vi "Cal11-RunMeasurement.vi"(0 "String in":refnum<vi>, 1 "reference in":refnum<vi>, 2 "Results file output":path, 3 "Array 5":dbl[](array[numeric]), 4 "Array 10":dbl[](array[numeric]), 6 "Array in":dbl[](array[numeric]), 7 "Array 6":dbl[](array[numeric]), 8 "data mode":enum16{"Take new data point", "Refit Curve"}(ring), 9 "Array 11":dbl[](array[numeric]), 11 "-ve Ref Values":bool) -> (10 "Array 8":dbl[](array[numeric]), 12 "Array 7":dbl[](array[numeric]), 13 "Status Out":T1, 14 "Array 9":dbl[](array[numeric]), 15 "Array 4":dbl[](array[numeric]), 16 "Array 3":dbl[](array[numeric]), 17 "String":string, 18 "Sample of input signals":dbl[][](graph))   [LabVIEW 2016]
uses:
  Anemometry Sub Vis/Gen Trav/Multi_Run_Status.ctl
  Anemometry Sub Vis/Controls/Setup.ctl
  Anemometry Sub Vis/Controls/Post_Process.ctl
  Anemometry Sub Vis/Controls/Save_Data.ctl
  <vilib>/Analysis/baseanly.llb/Mean (DBL).vi
  Anemometry Sub Vis/Globals/Calib_global.vi
  Anemometry Sub Vis/Globals/Meas_global.vi
  Anemometry Sub Vis/Acquisition/PWA/PWAtasksGLOBAL.vi
  <vilib>/Analysis/NI_AALBase.lvlib
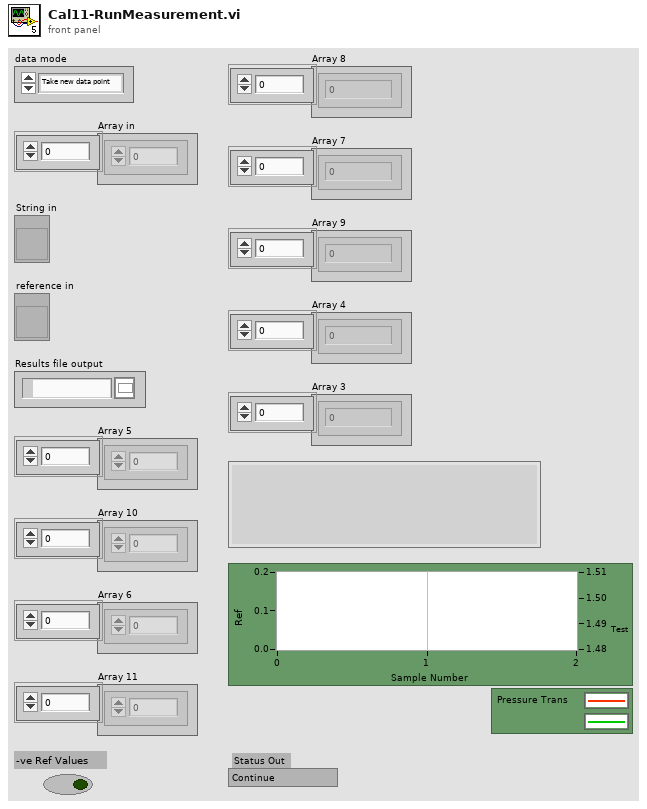
[diagram p1: front panel]
types:
  T1 = typedef "Multi_Run_Status.ctl" = enum16{"Continue", "Jump to Next Point", "Jump to Next Row", "Jump To Fall Back", "Terminate Run"}
  T2 = typedef "Cal_Inst_type.ctl" = enum16{"Propeller anemometer", "Pressure Transducer", "Hot wire", "Cross wire velocity", "Cross wire angle", "Generic Linear", "Generic Polynomial", "Generic BackPoly", "Fast FID", "Thermocouple", "Cold wire", "Pulsed Wire"}
  T3 = typedef "Ref_Inst_type.ctl" = enum16{"Propellor anemometer", "Pressure Transducer", "Raw voltage", "Pitot-static tube", "Preston tube", "Generic Linear", "Generic Polynomial", "Thermocouple", "LDA", "Enter Value", "ADAM Channel"}
  T4 = cluster{"2nd Ref type":T3, "2nd inst present":bool}
  T5 = typedef "Save_Data.ctl" = enum16{"Save No Data", "Save Data"}
  T6 = typedef "Post_Process.ctl" = enum16{"Take New Data", "Post Process Raw Data File"}
  T7 = typedef "Setup.ctl" = enum16{"Run Program", "Show Setup", "Save Current Setup", "Setup Front Panel"}
  T8 = typedef "Analysis_info_cluster.ctl" = cluster{"Colour":u32, "Inst type":T9, "Inst name":string, "Symbol":string, "Code name":string, "Extra Info":string, "Inst Array":T10, "Extra Titles":string[], "Extra Values":string[], "U":dbl, "u^2":dbl, "u^3":dbl, "u^4":dbl, "Skew_u":dbl, "Kurt_u":dbl, "Sd Error in Mean":dbl, "% u'/U":dbl, "X":dbl, "Y":dbl, "Z":dbl, "Timescale integral Estimate":dbl, "Sd Error in Variance":dbl, "Calib File":path, "Calib Constants":dbl[], "Output Position":bool, "Full Stats":bool, "Av Sampling Rate":dbl, "Av No of Samples":dbl, "Total Meas Time (s)":dbl, "ADAM Ch Name":string, "Max value":dbl, "Min value":dbl}
  T9 = typedef "Inst_type.ctl" = enum16{"Propeller anemometer", "Raw voltage", "Pressure Transducer", "Pitot-static tube", "Preston tube", "Hot wire", "Cross wire 1", "Cross wire 2", "Generic Linear", "Generic Polynomial", "Generic BackPoly", "Fast FID", "Thermocouple", "Cold wire", "Pulsed Wire", "LDA Vel", "LDA Tran time", "LDA Arr time", "Microphone"}
  T10 = typedef "Instrument_Array.ctl" = enum16{"PWA", "LDA", "Analogue"}
  T11 = typedef "Time_Trace_Cluster.ctl" = cluster{"Weighting":dbl[], "Time (s)":dbl[], "Voltage":dbl[], "Eng Values":dbl[]}
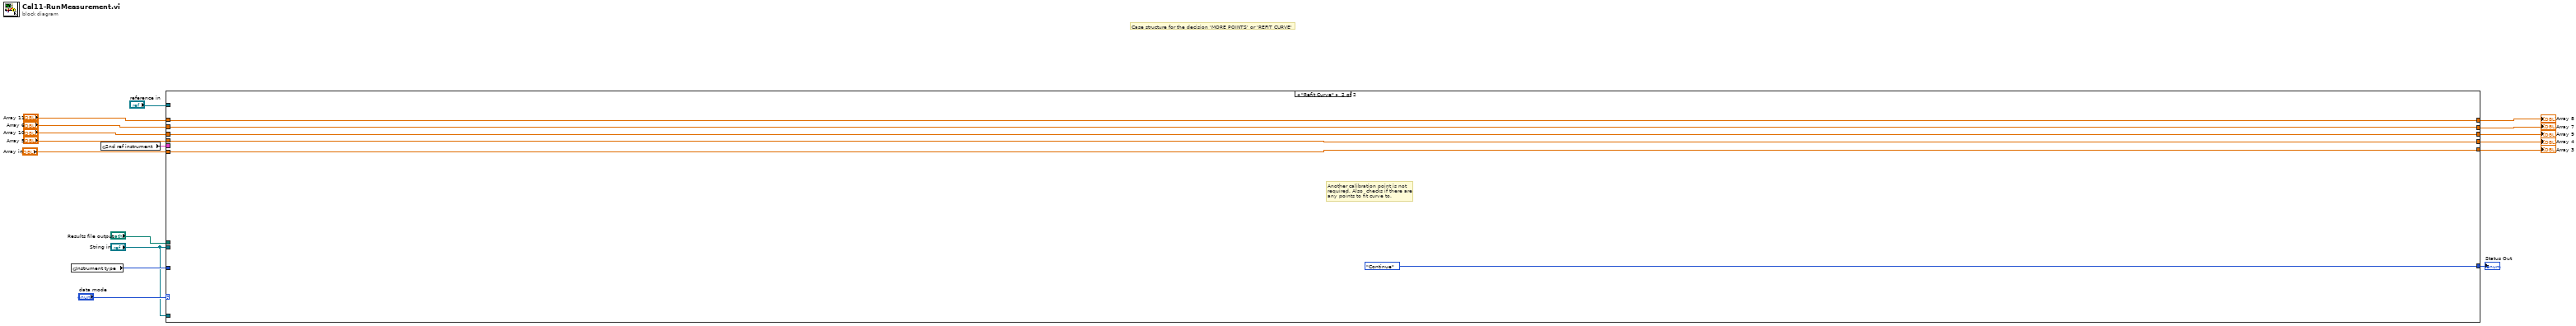
[diagram p0: block diagram]
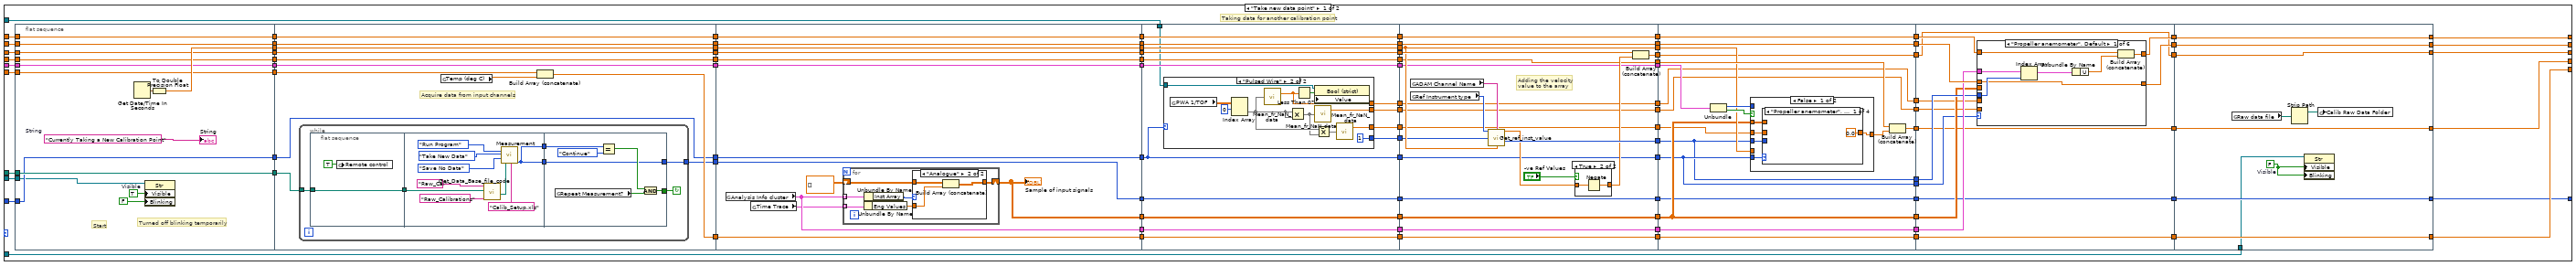
[diagram p2: hidden frame]
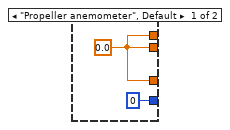
[diagram p4: hidden frame]
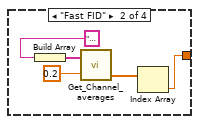
[diagram p6: hidden frame]
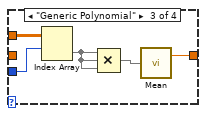
[diagram p7: hidden frame]
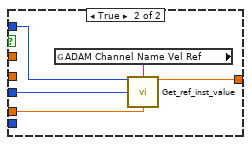
[diagram p9: hidden frame]
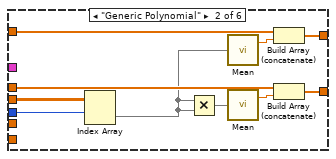
[diagram p10: hidden frame]
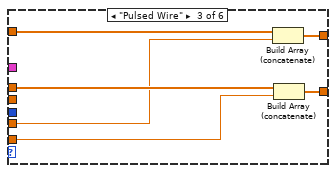
[diagram p11: hidden frame]
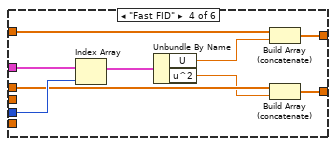
[diagram p12: hidden frame]
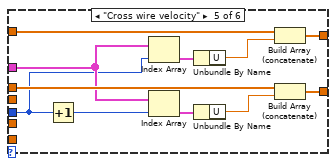
[diagram p13: hidden frame]
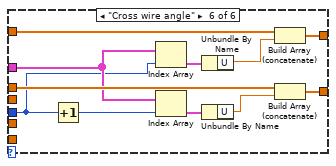
[diagram p14: hidden frame]
diagram:
  # "Case structure for the decision 'MORE POINTS' or 'REFIT CURVE'"
  n1 = global read "Calib_global.vi" "Instrument type"() -> (w16:T2)
  n2 = global read "Calib_global.vi" "2nd ref instrument"() -> (w11:T4)
  n3 = case shown="\"Refit Curve\"" "data mode" {
    tunnel: [w108 w362] -> w6
    tunnel: [w109 w358] -> w5
    tunnel: "Array 11" -> [w110 w362]
    tunnel: "Array 10" -> [w111 w358]
    tunnel: [w107 w361] -> w7
    tunnel: "Array 6" -> [w106 w361]
    tunnel: "Array 5" -> [w105 w360]
    tunnel: [w103 w360] -> w10
    tunnel: w11 -> [w104 _]
    tunnel: [w101 w359] -> w12
    tunnel: "Array in" -> [w102 w359]
    tunnel: "Results file output" -> [w100 _]
    tunnel: [w99 Multi_Run_Status."Continue" ("Status Out")] -> w13
    tunnel: w16 -> [w98 _]
    tunnel: "String in" -> [w20 _]
    tunnel: "reference in" -> [w19 _]
    tunnel: "String in" -> [w18 _]
    frame "Take new data point" {
      # "Taking data for another calibration point"
      # "Start"
      n4 = flat-sequence {
        tunnel: w110 -> [w122]
        tunnel: [w122] -> w97
        tunnel: w111 -> [w121]
        tunnel: [w121] -> w96
        tunnel: w106 -> [w120]
        tunnel: [w120] -> w95
        tunnel: w105 -> [w119]
        tunnel: [w119] -> w94
        tunnel: w104 -> [w118]
        tunnel: [w118] -> w93
        tunnel: w102 -> [w117]
        tunnel: [w117] -> w92
        tunnel: w100 -> [w116]
        tunnel: [w116] -> w91
        tunnel: w98 -> [w115]
        tunnel: [w115] -> w90
        tunnel: [w125] -> w89
        tunnel: w20 -> [w113]
        tunnel: w97 -> [w132]
        tunnel: [w132] -> w88
        tunnel: w96 -> [w131]
        tunnel: [w131] -> w87
        tunnel: w95 -> [w130]
        tunnel: [w130] -> w86
        tunnel: w94 -> [w129]
        tunnel: [w129] -> w85
        tunnel: w93 -> [w128]
        tunnel: [w128] -> w84
        tunnel: w92 -> [w137]
        tunnel: [w136] -> w83
        tunnel: w91 -> [w134]
        tunnel: [w135] -> w82
        tunnel: w90 -> [w127]
        tunnel: [w127] -> w81
        tunnel: w89 -> [w126]
        tunnel: [w126] -> w80
        tunnel: w88 -> [w170]
        tunnel: [w170] -> w79
        tunnel: w87 -> [w169]
        tunnel: [w169] -> w78
        tunnel: w86 -> [w168]
        tunnel: [w168] -> w77
        tunnel: w85 -> [w167]
        tunnel: [w167] -> w76
        tunnel: w84 -> [w166]
        tunnel: [w166] -> w75
        tunnel: w83 -> [w165]
        tunnel: [w165] -> w74
        tunnel: w82 -> [w164]
        tunnel: [w164] -> w73
        tunnel: w81 -> [w163]
        tunnel: [w163] -> w72
        tunnel: w80 -> [w162]
        tunnel: [w162] -> w71
        tunnel: [w173] -> w70
        tunnel: [w161] -> w69
        tunnel: w79 -> [w195]
        tunnel: [w195] -> w68
        tunnel: w78 -> [w194]
        tunnel: [w194] -> w67
        tunnel: w77 -> [w193]
        tunnel: [w193] -> w66
        tunnel: w76 -> [w192]
        tunnel: [w192] -> w65
        tunnel: w75 -> [w191]
        tunnel: [w191] -> w64
        tunnel: w74 -> [w190]
        tunnel: [w190] -> w63
        tunnel: w73 -> [w189]
        tunnel: [w189] -> w62
        tunnel: w72 -> [w198]
        tunnel: [w198] -> w61
        tunnel: w71 -> [w188]
        tunnel: [w188] -> w60
        tunnel: w70 -> [w187]
        tunnel: [w187] -> w59
        tunnel: w69 -> [w186]
        tunnel: [w186] -> w58
        tunnel: [w199] -> w57
        tunnel: [w197] -> w56
        tunnel: [w196] -> w55
        tunnel: [w185] -> w54
        tunnel: w19 -> [w184]
        tunnel: w68 -> [w224]
        tunnel: [w224] -> w53
        tunnel: [w234] -> w52
        tunnel: w67 -> [w233]
        tunnel: w66 -> [w223]
        tunnel: [w223] -> w51
        tunnel: w65 -> [w222]
        tunnel: [w222] -> w50
        tunnel: w64 -> [w221]
        tunnel: [w221] -> w49
        tunnel: w63 -> [w220]
        tunnel: [w220] -> w48
        tunnel: w62 -> [w219]
        tunnel: [w219] -> w47
        tunnel: w61 -> [w218]
        tunnel: [w218] -> w46
        tunnel: [w231] -> w45
        tunnel: w60 -> [w232]
        tunnel: [w232] -> w44
        tunnel: w59 -> [w217]
        tunnel: [w217] -> w43
        tunnel: w58 -> [w216]
        tunnel: [w216] -> w42
        tunnel: w57 -> [w227]
        tunnel: w56 -> [w215]
        tunnel: [w215] -> w41
        tunnel: w55 -> [w214]
        tunnel: [w214] -> w40
        tunnel: w54 -> [w213]
        tunnel: [w213] -> w39
        tunnel: w53 -> [w246]
        tunnel: [w246] -> w38
        tunnel: w52 -> [w245]
        tunnel: [w245] -> w37
        tunnel: w51 -> [w244]
        tunnel: [w244] -> w36
        tunnel: w50 -> [w253]
        tunnel: [w252] -> w35
        tunnel: w49 -> [w251]
        tunnel: w48 -> [w243]
        tunnel: [w243] -> w34
        tunnel: w47 -> [w239]
        tunnel: [w239] -> w33
        tunnel: w46 -> [w248]
        tunnel: [w248] -> w32
        tunnel: w45 -> [w238]
        tunnel: w44 -> [w250]
        tunnel: w43 -> [w242]
        tunnel: [w242] -> w31
        tunnel: [w238] -> w30
        tunnel: w42 -> [w249]
        tunnel: [w249] -> w29
        tunnel: w41 -> [w241]
        tunnel: [w241] -> w28
        tunnel: w40 -> [w240]
        tunnel: [w240] -> w27
        tunnel: w39 -> [w247]
        tunnel: w38 -> [w292]
        tunnel: w37 -> [w282]
        tunnel: [w282] -> w26
        tunnel: [w291] -> w25
        tunnel: [w290] -> w24
        tunnel: w36 -> [w289]
        tunnel: w35 -> [w281]
        tunnel: [w281] -> w23
        tunnel: w34 -> [w280]
        tunnel: [w280] -> w22
        tunnel: w33 -> [w279]
        tunnel: [w279] -> w21
        tunnel: w32 -> [w285]
        tunnel: w31 -> [w288]
        tunnel: w30 -> [w287]
        tunnel: w29 -> [w286]
        tunnel: w28 -> [w284]
        tunnel: w27 -> [w283]
        tunnel: [w354] -> w109
        tunnel: w26 -> [w354]
        tunnel: [w353] -> w108
        tunnel: w25 -> [w353]
        tunnel: [w352] -> w107
        tunnel: w24 -> [w352]
        tunnel: [w351] -> w103
        tunnel: w23 -> [w351]
        tunnel: [w350] -> w101
        tunnel: w22 -> [w350]
        tunnel: [w349] -> w99
        tunnel: w21 -> [w349]
        tunnel: w18 -> [w347]
        frame #0 {
          w123 = TRUE  # Visible
          w114 = "Currently Taking a New Calibration Point"  # String
          # "Turned off blinking temporarily"
          n5 = Get Date/Time In Seconds() -> (seconds since 1Jan1904=w124:timestamp)
          n6 = property on="Property Node" class="Str"(reference=w113, "Visible"=w123, "Blinking"=FALSE) -> ()  [unwired: 1 in, 2 out]
          n7 = To Double Precision Float(number=w124) -> (double precision float=w125:dbl)
          "String" <- w114
        }
        frame #1 {
          # "Acquire data from input channels"
          n8 = while {
            tunnel: [w143] -> w135
            tunnel: w134 -> [w142]
            stop <- w141 continue-if-true
            n9 = flat-sequence {
              tunnel: w142 -> [w144]
              tunnel: [w144] -> w140
              tunnel: [w147] -> w139
              tunnel: w140 -> [w151]
              tunnel: [w147] -> w138
              tunnel: [w155] -> w143
              tunnel: w139 -> [w155]
              tunnel: [w157] -> w141
              tunnel: w138 -> [w156]
              frame #0 {
                n10 = global write "Meas_global.vi" "Remote control"(TRUE ("Remote control")) -> ()
              }
              frame #1 {
                n11 = call "Get_Data_Base_file_code.vi"("Data Type"="Raw_Calibrations", "Results Filename"=w151, "Short_Name"="Raw_Cal" ("Data Type")) -> ("Raw Data File Name"=w148:path)  [unwired: 1 in, 3 out]
                n12 = call "Measurement.vi"("setup"=Setup."Run Program", "Post Process"=Post_Process."Take New Data", "File"=Save_Data."Save No Data", "Raw data file"=w148, "Setup filename"="Calib_Setup.xls") -> ("Status Out"=w147:T1)  [unwired: 2 in, 12 out]
              }
              frame #2 {
                n13 = global read "Meas_global.vi" "Repeat Measurement?"() -> (w158:bool)
                n14 = Equal?(x=w156, y=Multi_Run_Status."Continue" ("Status Out")) -> (x = y?=w159:bool)
                n15 = And(x=w159, y=w158) -> (x .and. y?=w157:bool)
              }
            }
          }
          n16 = global read "Calib_global.vi" "Temp (deg C)"() -> (w133:dbl)
          n17 = Build Array (concatenate)(w137, w133) -> (w136:dbl[])
        }
        frame #2 {
          n18 = global read "Meas_global.vi" "Analysis Info cluster"() -> (w173:T8[])
          n19 = global read "Meas_global.vi" "Time Trace"() -> (w171:T11[])
          n20 = for {
            tunnel: w173 -> [w179] mode=indexing
            shift-right: [w176] -> w161
            shift-left: dbl[][] [] -> [w177]
            tunnel: w171 -> [w175] mode=indexing
            n21 = Unbundle By Name(w175) -> ("Eng Values"=w174:dbl[])
            n22 = Unbundle By Name(w179) -> ("Inst Array"=w178:T10)
            n23 = case shown="\"Analogue\"" w178 {
              tunnel: w177 -> [w180 w183]
              tunnel: w174 -> [_ w182]
              tunnel: [w180 w181] -> w176
              frame "PWA", Default {
              }
              frame "Analogue" {
                n24 = Build Array (concatenate)(w183, w182) -> (w181:dbl[][])
              }
            }
          }
          "Sample of input signals" <- w161
        }
        frame #3 {
          n25 = case shown="\"Pulsed Wire\"" w198 {
            tunnel: [0 ("Index in") 1 ("Index in")] -> w199
            tunnel: [w200 w204] -> w197
            tunnel: [w200 w208] -> w196
            tunnel: [w200 w207] -> w185
            tunnel: w184 -> [_ w202]
            frame "Propeller anemometer", Default {
              w200 = 0.0 ("mean")
            }
            frame "Pulsed Wire" {
              n26 = global read "PWAtasksGLOBAL.vi" "PWA 1/TOF"() -> (w211:dbl[][])
              n27 = Index Array(array=w211, index (row)=0) -> (element=w209:dbl[])  [unwired: 1 in]
              n28 = call "Mean_fr_NaN_data.vi"("Data"=w209) -> ("Mean value"=w204:dbl)  [unwired: 1 out]
              n29 = Multiply(x=w209, y=w209) -> (x*y=w206:dbl[])
              n30 = Less Than 0?(x=w204) -> (x < 0?=w203:bool)
              n31 = property class="Bool (strict)"(reference=w202, "Value"=w203) -> ()  [unwired: 1 in, 2 out]
              n32 = call "Mean_fr_NaN_data.vi"("Data"=w206) -> ("Mean value"=w208:dbl)  [unwired: 1 out]
              n33 = Multiply(x=w209, y=w206) -> (x*y=w205:dbl[])
              n34 = call "Mean_fr_NaN_data.vi"("Data"=w205) -> ("Mean value"=w207:dbl)  [unwired: 1 out]
            }
          }
        }
        frame #4 {
          # "Adding the velocity\nvalue to the array"
          n35 = global read "Calib_global.vi" "ADAM Channel Name"() -> (w225:string)
          n36 = global read "Calib_global.vi" "Ref Instrument type"() -> (w230:T3)
          n37 = call "Get_ref_inst_value.vi"("Ref Instrument type"=w230, "ADAM Channel Name"=w225, "Index in"=w227, "Start time"=w232) -> ("Ref Value"=w229:dbl, "Index out"=w231:i32)  [unwired: 3 in, 7 out]
          n38 = case shown="True" "-ve Ref Values" {
            tunnel: w229 -> [w235 w237]
            tunnel: [w235 w236] -> w228
            frame False {
            }
            frame True {
              n39 = Negate(x=w237) -> (-x=w236:dbl)
            }
          }
          n40 = Build Array (concatenate)(w233, w228) -> (w234:dbl[])
        }
        frame #5 {
          n41 = Unbundle(w251) -> ("2nd Ref type"=w255:T3, "2nd inst present"=w254:bool)
          n42 = case shown="False" w254 {
            tunnel: w238 -> [w261 w275]
            tunnel: [w259 w276] -> w256
            tunnel: w255 -> [_ w277]
            tunnel: w250 -> [_ w278]
            tunnel: w249 -> [w260 _]
            tunnel: w248 -> [w258 _]
            tunnel: w247 -> [w257 _]
            frame False {
              n43 = case shown="\"Propeller anemometer\", Default" w258 {
                tunnel: w261 -> [_ _ w272 _]
                tunnel: w260 -> [_ _ w271 _]
                tunnel: [0.0 ("mean") w263 w269 w273] -> w259
                tunnel: w257 -> [_ _ _ w273]
                frame "Propeller anemometer", Default {
                }
                frame "Fast FID" {
                  n44 = Build Array("GMU:Source:ppm/%Density") -> (w266:string[])
                  n45 = call "Get_Channel_averages.vi"("Desired Ch Names"=w266, "Averaging time (mins)"=0.2) -> ("number"=w264:dbl[])  [unwired: 1 in, 2 out]
                  n46 = Index Array(array=w264) -> (element=w263:dbl)  [unwired: 1 in]
                }
                frame "Generic Polynomial" {
                  n47 = Index Array(array=w271, index (row)=w272) -> (element=w268:dbl[])  [unwired: 1 in]
                  n48 = Compound Arithmetic op=MULTIPLY(w268, w268, w268) -> (w270:dbl[])
                  n49 = call-poly <vilib>:"Mean.vi"("X"=w270) -> ("mean"=w269:dbl)  [unwired: 1 out]
                }
                frame "Pulsed Wire" {
                }
              }
            }
            frame True {
              n50 = global read "Calib_global.vi" "ADAM Channel Name Vel Ref"() -> (w274:string)
              n51 = call "Get_ref_inst_value.vi"("Ref Instrument type"=w277, "ADAM Channel Name"=w274, "Index in"=w275, "Start time"=w278) -> ("Ref Value"=w276:dbl)  [unwired: 4 in, 7 out]
            }
          }
          n52 = Build Array (concatenate)(w253, w256) -> (w252:dbl[])
        }
        frame #6 {
          n53 = case shown="\"Propeller anemometer\", Default" w285 {
            tunnel: w292 -> [w297 w307 w314 w322 w334 w345]
            tunnel: [w298 w308 w315 w323 w335 w346] -> w291
            tunnel: w289 -> [w296 w306 w313 w318 w333 w344]
            tunnel: [w296 w305 w312 w316 w332 w343] -> w290
            tunnel: w288 -> [w294 _ _ w320 w328 w339]
            tunnel: w287 -> [w299 w309 _ w324 w326 w337]
            tunnel: w286 -> [_ w304 _ _ _ _]
            tunnel: w284 -> [_ _ w311 _ _ _]
            tunnel: w283 -> [_ _ w310 _ _ _]
            frame "Propeller anemometer", Default {
              n54 = Index Array(array=w294, index=w299) -> (element=w295:T8)
              n55 = Unbundle By Name(w295) -> ("U"=w293:dbl)
              n56 = Build Array (concatenate)(w297, w293) -> (w298:dbl[])
            }
            frame "Generic Polynomial" {
              n57 = Index Array(array=w304, index (row)=w309) -> (element=w301:dbl[])  [unwired: 1 in]
              n58 = Multiply(x=w301, y=w301) -> (x*y=w300:dbl[])
              n59 = call-poly <vilib>:"Mean.vi"("X"=w301) -> ("mean"=w303:dbl)  [unwired: 1 out]
              n60 = call-poly <vilib>:"Mean.vi"("X"=w300) -> ("mean"=w302:dbl)  [unwired: 1 out]
              n61 = Build Array (concatenate)(w307, w303) -> (w308:dbl[])
              n62 = Build Array (concatenate)(w306, w302) -> (w305:dbl[])
            }
            frame "Pulsed Wire" {
              n63 = Build Array (concatenate)(w314, w311) -> (w315:dbl[])
              n64 = Build Array (concatenate)(w313, w310) -> (w312:dbl[])
            }
            frame "Fast FID" {
              n65 = Index Array(array=w320, index=w324) -> (element=w321:T8)
              n66 = Unbundle By Name(w321) -> ("U"=w319:dbl, "u^2"=w317:dbl)
              n67 = Build Array (concatenate)(w322, w319) -> (w323:dbl[])
              n68 = Build Array (concatenate)(w318, w317) -> (w316:dbl[])
            }
            frame "Cross wire velocity" {
              n69 = Increment(x=w326) -> (x+1=w325:i32)
              n70 = Index Array(array=w328, index=w326) -> (element=w331:T8)
              n71 = Index Array(array=w328, index=w325) -> (element=w330:T8)
              n72 = Unbundle By Name(w331) -> ("U"=w327:dbl)
              n73 = Unbundle By Name(w330) -> ("U"=w329:dbl)
              n74 = Build Array (concatenate)(w334, w327) -> (w335:dbl[])
              n75 = Build Array (concatenate)(w333, w329) -> (w332:dbl[])
            }
            frame "Cross wire angle" {
              n76 = Increment(x=w337) -> (x+1=w336:i32)
              n77 = Index Array(array=w339, index=w337) -> (element=w342:T8)
              n78 = Index Array(array=w339, index=w336) -> (element=w341:T8)
              n79 = Unbundle By Name(w342) -> ("U"=w338:dbl)
              n80 = Unbundle By Name(w341) -> ("U"=w340:dbl)
              n81 = Build Array (concatenate)(w345, w338) -> (w346:dbl[])
              n82 = Build Array (concatenate)(w344, w340) -> (w343:dbl[])
            }
          }
        }
        frame #7 {
          w348 = FALSE  # Visible
          n83 = global read "Meas_global.vi" "Raw data file"() -> (w356:path)
          n84 = Strip Path(path=w356) -> (stripped path=w355:path)  [unwired: 1 out]
          n85 = property on="Property Node" class="Str"(reference=w347, "Visible"=w348, "Blinking"=w348) -> ()  [unwired: 1 in, 2 out]
          n86 = global write "Calib_global.vi" "Calib Raw Data Folder"(w355) -> ()
        }
      }
    }
    frame "Refit Curve" {
      # "Another calibration point is not\nrequired. Also  checks if there are\nany points to fit curve to."
    }
  }
  "Status Out" <- w13
  "Array 3" <- w12
  "Array 4" <- w10
  "Array 7" <- w7
  "Array 8" <- w6
  "Array 9" <- w5
